vi "Select File.vi"(7 "Files Found":bool, 8 "error in (no error)":errorcluster, 9 "Current File in":i32, 10 "PREV":bool, 11 "NEXT":bool) -> (0 "error out":errorcluster, 1 "Current File out":i32)   [LabVIEW 2020]
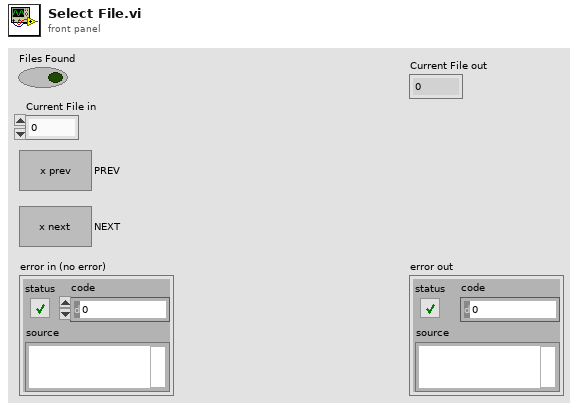
[diagram p1: front panel]
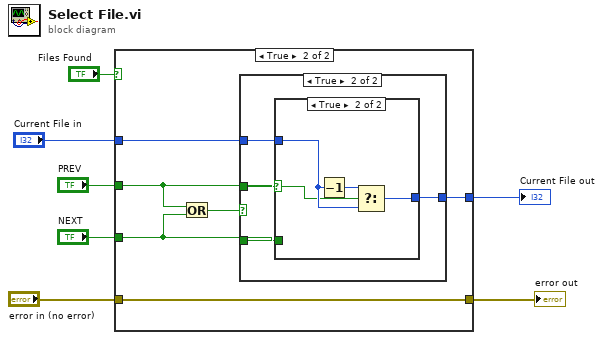
[diagram p0: block diagram]
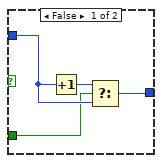
[diagram p4: hidden frame]
diagram:
  n1 = case shown="True" "Files Found" {
    tunnel: [w8 w10] -> w4
    tunnel: [w9 w15] -> w2
    tunnel: "Current File in" -> [w9 w14]
    tunnel: "error in (no error)" -> [w8 w10]
    tunnel: "NEXT" -> [_ w12]
    tunnel: "PREV" -> [_ w11]
    frame False {
    }
    frame True {
      n2 = Or(x=w11, y=w12) -> (x .or. y?=w13:bool)
      n3 = case shown="True" w13 {
        tunnel: [w16 w20] -> w15
        tunnel: w14 -> [w16 w19]
        tunnel: w11 -> [_ w18]
        tunnel: w12 -> [_ w17]
        frame False {
        }
        frame True {
          n4 = case shown="True" w18 {
            selector: w18 -> [_ w25]
            tunnel: [w24 w28] -> w20
            tunnel: w19 -> [w23 w27]
            tunnel: w17 -> [w21 _]
            frame False {
              n5 = Increment(x=w23) -> (x+1=w22:i32)
              n6 = Select(t=w22, s=w21, f=w23) -> (s? t:f=w24:i32)
            }
            frame True {
              n7 = Decrement(x=w27) -> (x-1=w26:i32)
              n8 = Select(t=w26, s=w25, f=w27) -> (s? t:f=w28:i32)
            }
          }
        }
      }
    }
  }
  "error out" <- w4
  "Current File out" <- w2
